vi "Dummy.vi"(8 "error in (no error)":errorcluster, 11 "Dummy in":refnum<class "Dummy.lvclass">) -> (0 "error out":errorcluster, 3 "Dummy out":refnum<class "Dummy.lvclass">)   [LabVIEW 2009, in "Dummy.lvclass"]
uses:
  Dummy.lvclass
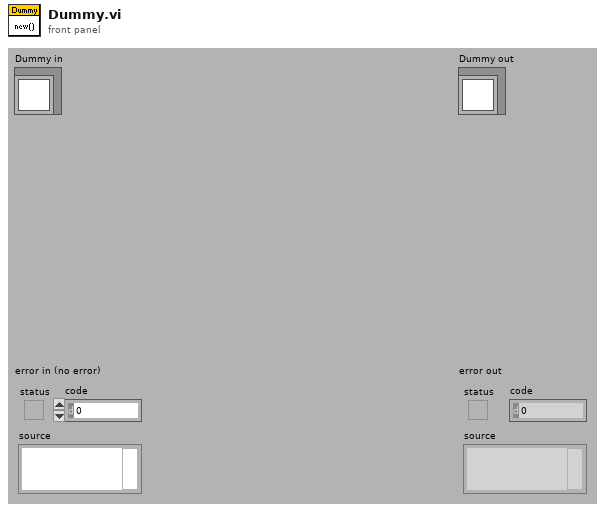
[diagram p1: front panel]
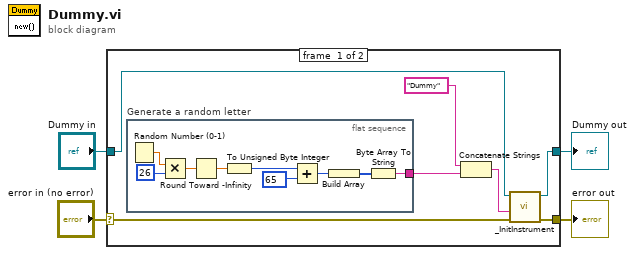
[diagram p0: block diagram]
diagram:
  n1 = case shown="No Error" "error in (no error)" {
    selector: "error in (no error)" -> [w9 w22]
    tunnel: [w8 w22] -> w3
    tunnel: [w10 w21] -> w1
    tunnel: "Dummy in" -> [w11 w21]
    frame #0 {
      n2 = flat-sequence "Generate a random letter" {
        tunnel: [w12] -> w6
        frame #0 {
          n3 = Random Number (0-1)() -> (number: 0 to 1=w19:dbl)
          n4 = Multiply(x=w19, y=u8 26) -> (x*y=w18:dbl)
          n5 = Round Toward -Infinity(1:w18) -> (0:w14:dbl)
          n6 = To Unsigned Byte Integer(number=w14) -> (unsigned 8bit integer=w13:u8)
          n7 = Add(x=w13, y=u8 65) -> (x+y=w16:u8)
          n8 = Build Array(w16) -> (w15:u8[])
          n9 = Byte Array To String(unsigned byte array=w15) -> (string=w12:string)
        }
      }
      n10 = Concatenate Strings("Dummy", w6) -> (w7:string)
      n11 = call-dynamic "_InitInstrument.vi"("error in (no error)"=w9, "Name"=w7, "Instrument in"=w11) -> ("error out"=w8:errorcluster, "Instrument out"=w10:refnum<class "Dummy.lvclass">)  [unwired: 3 in, 4 out]
    }
    frame #1 {
    }
  }
  "error out" <- w3
  "Dummy out" <- w1
